vi "wave.vi"   [LabVIEW 2012]
uses:
  <vilib>/addons/internet/NI_InternetTK_Core_VIs.lvlib
  <vilib>/addons/internet/NI_InternetTK_Common_VIs.lvlib
types:
  T1 = typedef "CGI Connection Info.ctl" = cluster{"name":string, "type":T2, "session":T3}
  T2 = typedef "CGI Request Type.ctl" = enum16{"cgi", ".spool first", ".spool", ".spool last"}
  T3 = typedef "HTTP Session.ctl" = refnum<k1>
  T4 = typedef "NI_FTP.lvlib/Keyed Array.ctl" = cluster{"keys":string[], "values":string[]}
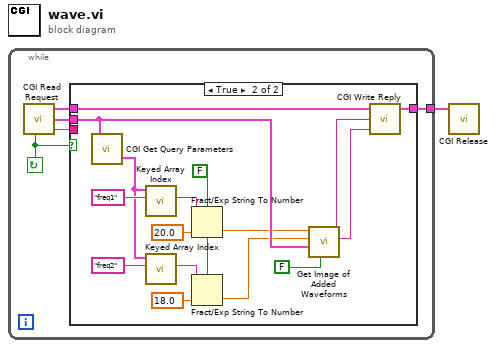
[diagram p0: block diagram]
diagram:
  n1 = while {
    tunnel: [w5] -> w1
    stop <- w4 continue-if-true
    n2 = call <vilib>:"CGI Read Request.vi"() -> ("valid request?"=w4:bool, "cgi connection info"=w6:T1, "env"=w3:T4, "content"=w2:string)  [unwired: 4 in]
    n3 = case shown="True" w4 {
      tunnel: [w7 w23] -> w5
      tunnel: w6 -> [w7 w22]
      tunnel: w3 -> [_ w14]
      tunnel: w2 -> [_ _]
      frame False {
      }
      frame True {
        w8 = FALSE ("use system decimal point (T)")
        n4 = call <vilib>:"CGI Get Query Parameters.vi"("env"=w14) -> ("query params"=w15:T4)  [unwired: 2 out]
        n5 = call <vilib>:"Keyed Array Index.vi"("key"="freq1", "array in"=w15) -> ("value"=w20:string)  [unwired: 3 in, 2 out]
        n6 = call <vilib>:"Keyed Array Index.vi"("key"="freq2", "array in"=w15) -> ("value"=w17:string)  [unwired: 3 in, 2 out]
        n7 = Fract/Exp String To Number(use system decimal point (T)=w8, string=w20, default (0 dbl)=20.0) -> (number=w13:dbl)  [unwired: 1 in, 1 out]
        n8 = Fract/Exp String To Number(use system decimal point (T)=w8, string=w17, default (0 dbl)=18.0) -> (number=w12:dbl)  [unwired: 1 in, 1 out]
        n9 = call "Get Image of Added Waveforms.vi"("close if closed (T)"=FALSE, "env"=w14, "Cycles 2"=w12, "Cycles 1"=w13) -> ("content"=w10:string, "content header"=w11:string)  [unwired: 5 in, 1 out]
        n10 = call <vilib>:"CGI Write Reply.vi"("content"=w10, "header"=w11, "cgi connection info"=w22) -> ("cgi connection info out"=w23:T1)  [unwired: 2 in]
      }
    }
  }
  n11 = call <vilib>:"CGI Release.vi"("cgi connection info"=w1) -> ()  [unwired: 5 in]
